vi "AfterPage2_GenCD.vi"(10 "MetaDataObj":refnum<class "MetaDataObj.lvclass">, 11 "User Project":refnum<vi>) -> ()   [LabVIEW 2015, in "NIVS_Consolidated_CDW_MetaDataObj.lvclass"]
uses:
  NIVS_Consolidated_CDW_MetaDataObj.lvclass
  <resource>/dialog/NewProjectWizard/MetaDataObj/MetaDataObj.lvclass
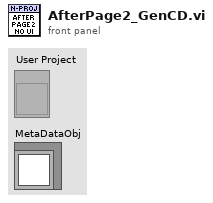
[diagram p1: front panel]
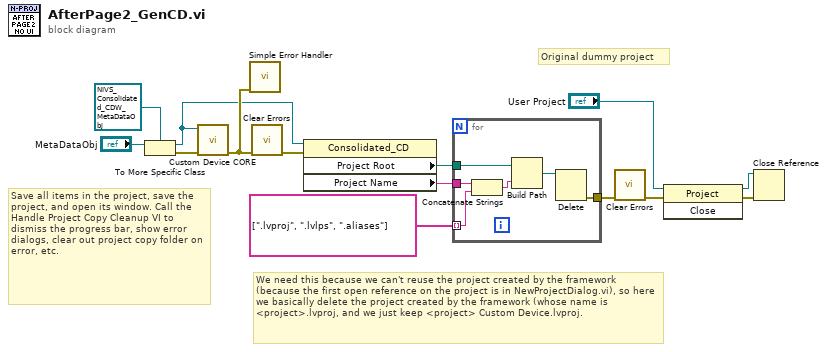
[diagram p0: block diagram]
diagram:
  # "Original dummy project"
  # "We need this because we can't reuse the project created by the framework (because the first open reference on the project is in NewProjectDialog.vi), so here we basically delete the project created by the framework (whose name is <project>.lvproj, and we just keep <project> Custom Device.lvproj."
  # "Save all items in the project, save the project, and open its window. Call the Handle Project Copy Cleanup VI to dismiss the progress bar, show error dialogs, clear out project copy folder on error, etc."
  n1 = To More Specific Class(target class=refnum<class "NIVS_Consolidated_CDW_MetaDataObj.lvclass"> refnum ("NIVS_CDW_MetaDataObj.lvclass"), reference="MetaDataObj") -> (specific class reference=w1:refnum<class "NIVS_Consolidated_CDW_MetaDataObj.lvclass">, error out=w12:errorcluster)  [unwired: 1 in]
  n2 = call "Custom Device CORE.vi"("error in (no error)"=w12, "CDW_MetaDataObj"=w1) -> ("error out"=w2:errorcluster)  [unwired: 9 in]
  n3 = call <vilib>:"Simple Error Handler.vi"("error in (no error)"=w2) -> ()  [unwired: 4 in, 5 out]
  n4 = call <vilib>:"Clear Errors.vi"("error in (no error)"=w2) -> ("error out"=w3:errorcluster)  [unwired: 5 in, 1 out]
  n5 = property class="Consolidated_CD"(reference=w1, error in=w3) -> ("Project Root"=w11:path, "Project Name"=w10:string)  [unwired: 2 out]
  n6 = for {
    tunnel: w11 -> [w20]
    tunnel: w10 -> [w19]
    tunnel: string[] [".lvproj", ".lvlps", ".aliases"] -> [w18] mode=indexing
    tunnel: [w15] -> w8
    n7 = Concatenate Strings(w19, w18) -> (w17:string)
    n8 = Build Path(base path=w20, name or relative path=w17) -> (appended path=w16:path)
    n9 = Delete(path (use dialog)=w16) -> (error out=w15:errorcluster)  [unwired: 4 in, 2 out]
  }
  n10 = call <vilib>:"Clear Errors.vi"("error in (no error)"=w8) -> ("error out"=w7:errorcluster)  [unwired: 5 in, 1 out]
  n11 = invoke class="Project" method="Close"(reference="User Project", error in=w7) -> (reference out=w4:refnum<vi>, error out=w5:errorcluster)  [unwired: 1 in, 1 out]
  n12 = Close Reference(reference=w4, error in (no error)=w5) -> ()  [unwired: 1 out]
